vi "Start.vi"(8 "error in (no error)":errorcluster, 11 "FolloWin in":refnum<class "FolloWin.lvclass">) -> (0 "error out":errorcluster, 3 "FolloWin out":refnum<class "FolloWin.lvclass">)   [LabVIEW 2023, in "FolloWin.lvclass"]
doc: "Runs FolloWin.vi if it is not already running."
uses:
  FolloWin.lvclass
  FolloWin.lvclass/FolloWin.ctl
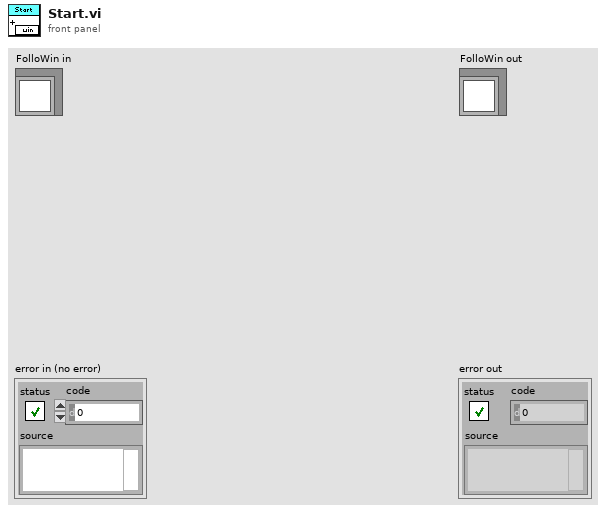
[diagram p1: front panel]
types:
  T1 = enum32{"Bad", "Idle", "Run top level", "Running"}
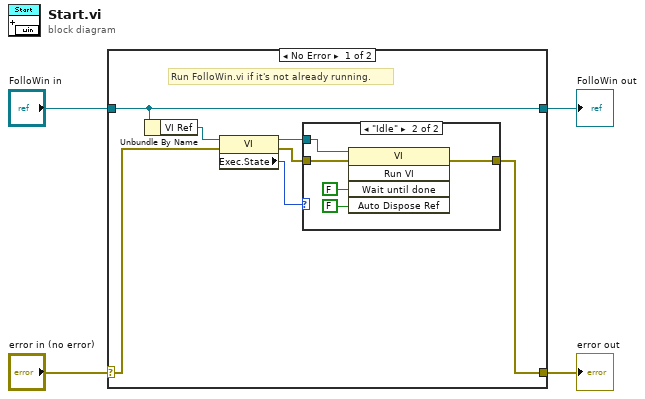
[diagram p0: block diagram]
diagram:
  n1 = case shown="No Error" "error in (no error)" {
    selector: "error in (no error)" -> [w6 w19]
    tunnel: [w10 w19] -> w3
    tunnel: [w11 w18] -> w1
    tunnel: "FolloWin in" -> [w11 w18]
    frame No Error {
      # "Run FolloWin.vi if it's not already running."
      n2 = Unbundle By Name(w11) -> ("VI Ref"=w9:refnum<vi>)
      n3 = property on="Property Node" class="VI"(reference=w9, error in=w6) -> (reference out=w7:refnum<vi>, error out=w5:errorcluster, "Exec.State"=w8:T1)
      n4 = case shown="\"Idle\"" w8 {
        tunnel: w5 -> [w12 w15]
        tunnel: [w12 w14] -> w10
        tunnel: w7 -> [_ w13]
        frame Default {
        }
        frame "Idle" {
          n5 = invoke on="Invoke Node" class="VI" method="Run VI"(reference=w13, error in=w15, "Wait until done"=FALSE ("Wait Until Done"), "Auto Dispose Ref"=FALSE ("Auto Dispose Reference")) -> (error out=w14:errorcluster)  [unwired: 1 in, 4 out]
        }
      }
    }
    frame Error {
    }
  }
  "error out" <- w3
  "FolloWin out" <- w1
